vi "Scan field at certain temp with SR830 and PPMS.vi"() -> ()   [LabVIEW 2019]
uses:
  <vilib>/Utility/file.llb/Write Delimited Spreadsheet (DBL).vi
panel:
  out "Current Task":i32
  out "PPMS IP Address":string="127.0.0.1"
  in  "Instrument Type":i32(ring) items=["PPMS", "VersaLab", "DynaCool", "SVSM"]
  in  "Remote":bool
  in  "Folder":string
  out "appended path":path
  out "XY Graph":cluster{dbl[], dbl[]}(graph)={[100.0, 90.0, 80.0, 70.0, 60.0, 50.0, 40.0, 30.0, 20.0, 10.0, 0.0, -10.0, -20.0], [0.000776771, 0.00077701, 0.000776831, 0.000777368, 0.00077701, 0.000777069, 0.000776354, 0.000776831, 0.00077695, 0.00077701, 0.000776593, 0.000776473, 0.000776533, 0.000777368, 0.000776712, 0.000777069, 0.000776712, 0.000776831, 0.00077695, 0.000776414, 0.00077701, 0.000776712, 0.000777189, 0.000776831, 0.000776712, 0.000776771, 0.000777189, 0.000776533, 0.000776295, 0.000776473, 0.000776771, 0.00077695, 0.000776831]}
  in  "Task Table":string[][](table)
  in  "SR830 GPIB Addr":string
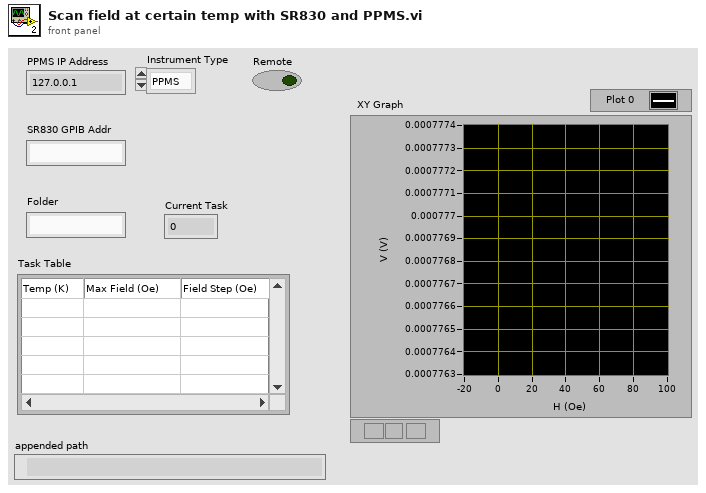
[diagram p1: front panel]
types:
  T1 = cluster{"Task Table[0]":string, "Task Table[1]":string, "Task Table[2]":string, "Task Table[3]":string, "Task Table[4]":string, "Task Table[5]":string, "Task Table[6]":string, "Task Table[7]":string, "Task Table[8]":string}
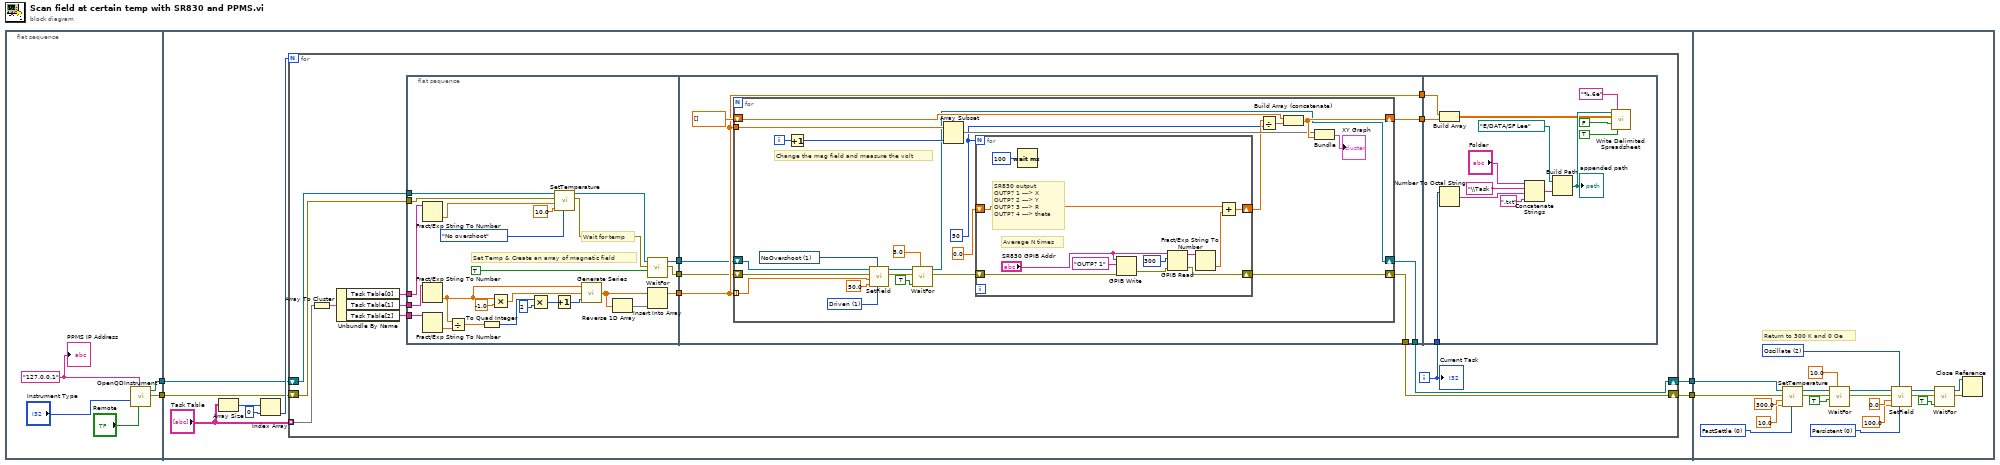
[diagram p0: block diagram]
diagram:
  n1 = flat-sequence {
    tunnel: [w6] -> w2
    tunnel: [w7] -> w1
    tunnel: [w11] -> w4
    tunnel: [w10] -> w3
    tunnel: w2 -> [w13]
    tunnel: w1 -> [w12]
    tunnel: w4 -> [w117]
    tunnel: w3 -> [w116]
    frame #0 {
      w8 = "127.0.0.1" ("IP Address")
      n2 = call "OpenQDInstrument.vi"("Remote"="Remote", "IP Address"=w8, "Instrument Type"="Instrument Type") -> ("error out"=w7:errorcluster, "Instrument Ref"=w6:refnum<k24>)  [unwired: 5 in]
      "PPMS IP Address" <- w8
    }
    frame #1 {
      n3 = Array Size(array="Task Table") -> (size(s)=w17:i32[])
      n4 = Index Array(array=w17, index=0) -> (element=w15:i32)
      n5 = for {
        N: w15 -> [_]
        tunnel: "Task Table" -> [w32] mode=indexing
        shift-right: [w18] -> w11
        shift-left: w13 -> [w21]
        shift-right: [w19] -> w10
        shift-left: w12 -> [w20]
        i -> [w24]
        n6 = Array To Cluster(array=w32) -> (cluster=w31:T1)
        n7 = Unbundle By Name(w31) -> ("Task Table[0]"=w28:string, "Task Table[1]"=w30:string, "Task Table[2]"=w29:string)
        n8 = flat-sequence {
          tunnel: [w34] -> w27
          tunnel: [w56] -> w23
          tunnel: [w53] -> w22
          tunnel: w20 -> [w39]
          tunnel: w21 -> [w40]
          tunnel: w28 -> [w44]
          tunnel: w29 -> [w51]
          tunnel: w30 -> [w52]
          tunnel: w27 -> [w62]
          tunnel: [w63] -> w26
          tunnel: [w62] -> w25
          tunnel: w23 -> [w61]
          tunnel: w22 -> [w60]
          tunnel: [w59] -> w19
          tunnel: [w58] -> w18
          tunnel: w24 -> [w107]
          tunnel: w25 -> [w110]
          tunnel: w26 -> [w111]
          frame #0 {
            # "Set Temp & Create an array of magnetic field"
            # "Wait for temp"
            n9 = Fract/Exp String To Number(string=w44) -> (number=w43:dbl)  [unwired: 3 in, 1 out]
            n10 = Fract/Exp String To Number(string=w52) -> (number=w36:dbl)  [unwired: 3 in, 1 out]
            n11 = Fract/Exp String To Number(string=w51) -> (number=w49:dbl)  [unwired: 3 in, 1 out]
            n12 = Divide(x=w36, y=w49) -> (x/y=w50:dbl)
            n13 = To Quad Integer(1:w50) -> (0:w48:i64)
            n14 = Multiply(x=w36, y=-1.0) -> (x*y=w37:dbl)
            n15 = Multiply(x=w48, y=i64 2) -> (x*y=w46:i64)
            n16 = Increment(x=w46) -> (x+1=w35:i64)
            n17 = call "SetTemperature.vi"("Approach"=enum16{"Fast Settle", "No overshoot"}."No overshoot" ("Approach Method"), "Rate"=10.0 ("Approach Rate( 0-20)"), "Temperature"=w43, "error in (no error)"=w39, "Instrument Ref In"=w40) -> ("error out"=w57:errorcluster, "Instrument Ref Out"=w54:refnum<k24>)  [unwired: 2 in, 1 out]
            n18 = call "Generate Series.vi"("Number of Points"=w35, "To"=w37, "From"=w36) -> ("Output Array"=w33:dbl[])
            n19 = Reverse 1D Array(array=w33) -> (reversed array=w45:dbl[])
            n20 = call "WaitFor.vi"("Wait For Temperature"=TRUE, "error in (no error)"=w57, "Instrument Ref In"=w54) -> ("error out"=w56:errorcluster, "Instrument Ref Out"=w53:refnum<k24>)  [unwired: 7 in]
            n21 = Insert Into Array(array=w33, new element=w45) -> (w34:dbl[])  [unwired: 1 in]
          }
          frame #1 {
            n22 = for {
              shift-right: [w81] -> w59
              shift-left: w61 -> [w76]
              shift-right: [w85] -> w63
              shift-left: dbl[] [] -> [w88]
              tunnel: w62 -> [w71] mode=indexing
              tunnel: w62 -> [w83]
              shift-right: [w65] -> w58
              shift-left: w60 -> [w73]
              i -> [w87]
              w72 = 1 items=["Linear", "NoOvershoot", "Oscillate"] ("Approach")
              w74 = 1 items=["Persistent", "Driven"] ("Mode")
              w78 = 50
              # "Change the mag field and measure the volt"
              n23 = Increment(x=w87) -> (x+1=w86:i32)
              n24 = call "SetField.vi"("Mode"=w74, "Approach"=w72, "Rate"=50.0, "Field"=w71, "error in (no error)"=w76, "Instrument Ref In"=w73) -> ("error out"=w69:errorcluster, "Instrument Ref Out"=w70:refnum<k24>)  [unwired: 1 in, 1 out]
              n25 = call "WaitFor.vi"("Delay"=5.0, "Wait For Field"=TRUE, "error in (no error)"=w69, "Instrument Ref In"=w70) -> ("error out"=w66:errorcluster, "Instrument Ref Out"=w65:refnum<k24>)  [unwired: 6 in]
              n26 = Array Subset(array=w83, length=w86) -> (w84:dbl[])  [unwired: 1 in]
              n27 = for {
                N: w78 -> [_]
                shift-right: [w92] -> w79
                shift-left: 0.0 -> [w91]
                shift-right: [w96] -> w81
                shift-left: w66 -> [w90]
                # "Average N times"
                # "SR830 output\nOUTP? 1 ---> X\nOUTP? 2 ---> Y\nOUTP? 3 ---> R\nOUTP? 4 ---> theta"
                n28 = Wait (ms)(milliseconds to wait=u32 100) -> ()  [unwired: 1 out]
                n29 = GPIB Write(0:"SR830 GPIB Addr", 1:"OUTP? 1" ("data"), 3:w90) -> (6:w97:errorcluster)  [unwired: 2 in, 1 out]
                n30 = GPIB Read(0:"SR830 GPIB Addr", 1:300 ("byte count"), 3:w97) -> (5:w95:string, 7:w96:errorcluster)  [unwired: 2 in, 1 out]
                n31 = Fract/Exp String To Number(string=w95) -> (number=w93:dbl)  [unwired: 3 in, 1 out]
                n32 = Add(x=w91, y=w93) -> (x+y=w92:dbl)
              }
              n33 = Divide(x=w79, y=w78) -> (x/y=w77:dbl)
              n34 = Build Array (concatenate)(w88, w77) -> (w85:dbl[])
              n35 = Bundle(w84, w85) -> (→"XY Graph":cluster{dbl[], dbl[]})  [unwired: 1 in]
            }
          }
          frame #2 {
            n36 = Build Array(w110, w111) -> (w109:dbl[][])
            n37 = Number To Octal String(2:w107) -> (0:w106:string)  [unwired: 1 in]
            n38 = Concatenate Strings("Folder", "\\Task " ("string"), w106, ".txt" ("string")) -> (w103:string)
            n39 = Build Path(base path=path "E:/DATA/SF Lee", name or relative path=w103) -> (appended path=w112:path)
            "appended path" <- w112
            n40 = call-poly <vilib>:"Write Delimited Spreadsheet.vi"("file path (dialog if empty)"=w112, "format (%.3f)"="%.6e", "2D data"=w109, "append to file? (new file:F)"=FALSE, "transpose? (no:F)"=TRUE) -> ()  [unwired: 9 in, 2 out]
          }
        }
        "Current Task" <- w24
      }
    }
    frame #2 {
      w121 = 2 items=["Linear", "NoOvershoot", "Oscillate"] ("Approach")
      w122 = 0 items=["Persistent", "Driven"] ("Mode")
      w133 = 0 items=["FastSettle", "NoOvershoot"] ("Approach")
      # "Return to 300 K and 0 Oe"
      n41 = call "SetTemperature.vi"("Approach"=w133, "Rate"=10.0 ("Approach Rate( 0-20)"), "Temperature"=300.0 ("Set Temperature"), "error in (no error)"=w116, "Instrument Ref In"=w117) -> ("error out"=w129:errorcluster, "Instrument Ref Out"=w130:refnum<k24>)  [unwired: 2 in, 1 out]
      n42 = call "WaitFor.vi"("Delay"=10.0, "Wait For Temperature"=TRUE, "error in (no error)"=w129, "Instrument Ref In"=w130) -> ("error out"=w123:errorcluster, "Instrument Ref Out"=w127:refnum<k24>)  [unwired: 6 in]
      n43 = call "SetField.vi"("Mode"=w122, "Approach"=w121, "Rate"=100.0, "Field"=0.0, "error in (no error)"=w123, "Instrument Ref In"=w127) -> ("error out"=w120:errorcluster, "Instrument Ref Out"=w119:refnum<k24>)  [unwired: 1 in, 1 out]
      n44 = call "WaitFor.vi"("Wait For Field"=TRUE, "error in (no error)"=w120, "Instrument Ref In"=w119) -> ("error out"=w114:errorcluster, "Instrument Ref Out"=w115:refnum<k24>)  [unwired: 7 in]
      n45 = Close Reference(reference=w115, error in (no error)=w114) -> ()  [unwired: 1 out]
    }
  }
